vi "BRig_dataTrial_iSpout.vi"() -> (2 "output_iSpout":i32)   [LabVIEW 2014]
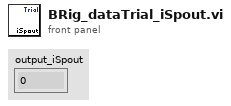
[diagram p1: front panel]
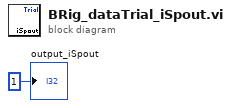
[diagram p0: block diagram]
diagram:
  "output_iSpout" <- 1 ("output_iBlock")
